vi "Update.vi"(8 "error in (no error)":errorcluster, 9 "Quem joga":string, 10 "Tabuleiro":T1, 11 "MatchData in":refnum<class "MatchData.lvclass">) -> (0 "error out":errorcluster, 3 "MatchData out":refnum<class "MatchData.lvclass">)   [LabVIEW 2018, in "MatchData.lvclass"]
uses:
  MatchData.lvclass
  controls/Tabuleiro.ctl
  MatchData.lvclass/MatchData.ctl
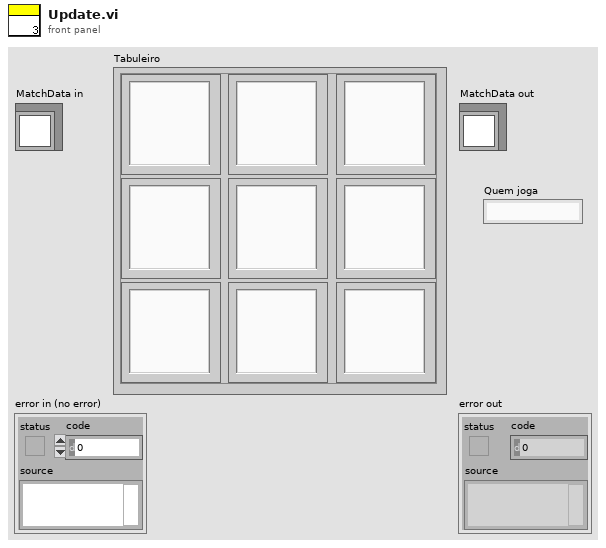
[diagram p1: front panel]
types:
  T1 = typedef "Tabuleiro.ctl" = cluster{"(0,0)":string, "(1,0)":string, "(0,1)":string, "(1,1)":string, "(2,0)":string, "(1,2)":string, "(2,2)":string, "(0,2)":string, "(2,1) ":string}
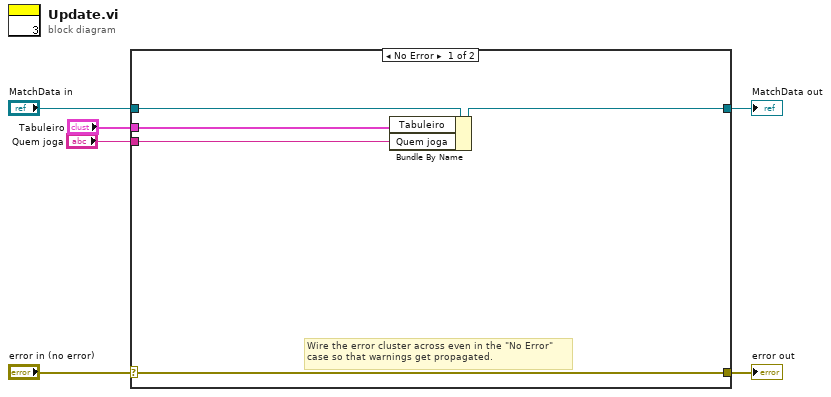
[diagram p0: block diagram]
diagram:
  n1 = case shown="No Error" "error in (no error)" {
    selector: "error in (no error)" -> [w10 w13]
    tunnel: [w10 w13] -> w5
    tunnel: [w9 w12] -> w3
    tunnel: "MatchData in" -> [w11 w12]
    tunnel: "Quem joga" -> [w8 _]
    tunnel: "Tabuleiro" -> [w7 _]
    frame No Error {
      # "Wire the error cluster across even in the \"No Error\"\ncase so that warnings get propagated."
      n2 = Bundle By Name(cluster=w11, "Tabuleiro"=w7, "Quem joga"=w8) -> (w9:refnum<class "MatchData.lvclass">)
    }
    frame Error {
    }
  }
  "error out" <- w5
  "MatchData out" <- w3
